vi "RT Driver VI.vi"(7 "Operation":T1, 11 "Device Reference in":T2 format="%.0x") -> (0 "Error Code":i32)   [LabVIEW 2015, in "Control Addon Engine.lvlib"]
uses:
  Control Addon Engine.lvlib
  <vilib>/NI Veristand/Custom Device API/Custom Device Item Ref.ctl
  <vilib>/NI Veristand/Custom Device API/Model Interface Driver VI Operation.ctl
  Types/RT Driver State Variables.ctl
  Types/RT Configuration.ctl
  Shared/Types/Gain Schedule.ctl
  Shared/Types/Compiled Settings.ctl
  Shared/Types/Compiled PID Settings.ctl
  <vilib>/NI Veristand/Custom Device API/Block Data Reference.ctl
  <vilib>/NI Veristand/Custom Device API/Data Reference.ctl
  Shared/Types/Compiled Industrial Settings.ctl
  Shared/Types/Compiled Industrial Parameters.ctl
  <vilib>/NI/NI VeriStand Inline Async API/_VS Inline Async API/VS Inline Async API/VS Inline Async API.lvclass
  <vilib>/NI Veristand/Custom Device API/NI VeriStand - Get Channel Values by Block Data Reference.vi
  <vilib>/addons/control/pid/pid.llb/PID Advanced (DBL Array).vi
  <vilib>/NI Veristand/Custom Device API/NI VeriStand - Set Channel Values by Block Data Reference.vi
  SubVIs/Get PID Gains from Schedule.vi
  SubVIs/Digital Debounce Filter.vi
  <vilib>/addons/control/pid/pid.llb/PID Parameter Manager (DBL Array).vi
  <vilib>/addons/control/pid/pid.llb/PID Derivative Action Buffered (DBL Array).vi
  <vilib>/addons/control/pid/pid.llb/PID Get Advanced Error (DBL Array).vi
  <vilib>/addons/control/pid/pid.llb/PID Integral Action Buffered (DBL Array).vi
  <vilib>/addons/control/pid/pid.llb/PID Resize 1D Array.vi
  <vilib>/addons/control/pid/pid.llb/PID Get Advanced Error (DBL).vi
  <vilib>/NI Veristand/Custom Device API/Global Data Refs.vi
  <vilib>/addons/control/pid/pid.llb/PID Gain Schedule.vi
  <vilib>/addons/control/pid/pid.llb/PID Gain Schedule (DBL).vi
  <vilib>/addons/control/pid/pid.llb/PID Output Rate Limiter.vi
  <vilib>/addons/control/pid/pid.llb/PID Output Rate Limiter (DBL Array).vi
  Shared/Control Addon Shared.lvlib
  <vilib>/NI VeriStand/Custom Device API/Custom Device API.lvlib
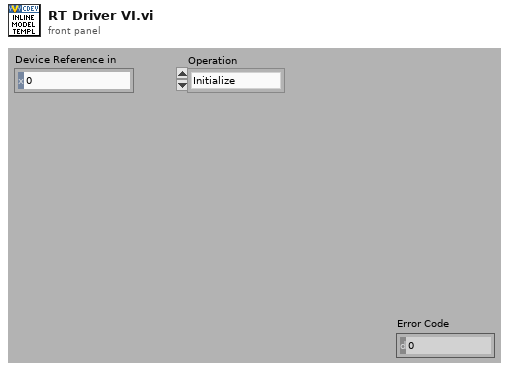
[diagram p1: front panel]
types:
  T1 = typedef "Custom Device API.lvlib/Model Interface Driver VI Operation.ctl" = enum16{"Initialize", "Start", "Execute Model", "Close"}
  T2 = typedef "Custom Device API.lvlib/Custom Device Item Ref.ctl" = u64
  T3 = typedef "Control Addon Engine.lvlib/RT Driver State Variables.ctl" = cluster{"Config":T4, "Init":bool, "Async":refnum<class "VS Inline Async API.lvclass">}
  T4 = typedef "Control Addon Engine.lvlib/RT Configuration.ctl" = cluster{"Parameter Refs":refnum<data-value>[], "Config":T5}
  T5 = typedef "Control Addon Shared.lvlib/Compiled Settings.ctl" = cluster{"PID Settings":T6, "Name":string, "Industrial Settings":T10}
  T6 = typedef "Control Addon Shared.lvlib/Compiled PID Settings.ctl" = cluster{"Gain Schedule":T7[], "Enable Live Updates":bool[], "output range":cluster{"output high":dbl, "output low":dbl}[], "setpoint range":cluster{"setpoint high":dbl, "setpoint low":dbl}[], "Write Refs":T8[], "Write Data":dbl[], "Read Refs":T8[], "Read Data":dbl[], "Control Loop Names":string[], "Enable Gain Scheduling":bool[], "Output Rate Limiter":dbl[], "dt":dbl, "setpoint high limit":dbl[], "setpoint low limit":dbl[], "output high limit":dbl[], "output low limit":dbl[]}
  T7 = typedef "Control Addon Shared.lvlib/Gain Schedule.ctl" = cluster{"Gain Schedule":cluster{"PID gains":cluster{"proportional gain (Kc)":dbl, "integral time (Ti, min)":dbl, "derivative time (Td, min)":dbl}, "max value":dbl}[]}
  T8 = typedef "Custom Device API.lvlib/Block Data Reference.ctl" = cluster{"Data Reference":T9, "Offset":u64, "Length":u64}
  T9 = typedef "Custom Device API.lvlib/Data Reference.ctl" = i32
  T10 = typedef "Control Addon Shared.lvlib/Compiled Industrial Settings.ctl" = cluster{"output range":cluster{"output high":dbl, "output low":dbl}[], "setpoint range":cluster{"setpoint high":dbl, "setpoint low":dbl}[], "Write Refs":T8[], "Write Data":dbl[], "Read Refs":T8[], "Read Data":dbl[], "Control Loop Names":string[], "Parameters":T11[], "Previous States":bool[], "Previous Counts":u64[]}
  T11 = typedef "Control Addon Shared.lvlib/Compiled Industrial Parameters.ctl" = cluster{"Enable Hysteresis":bool, "Hysteresis":dbl, "Minimum Switching":u64}
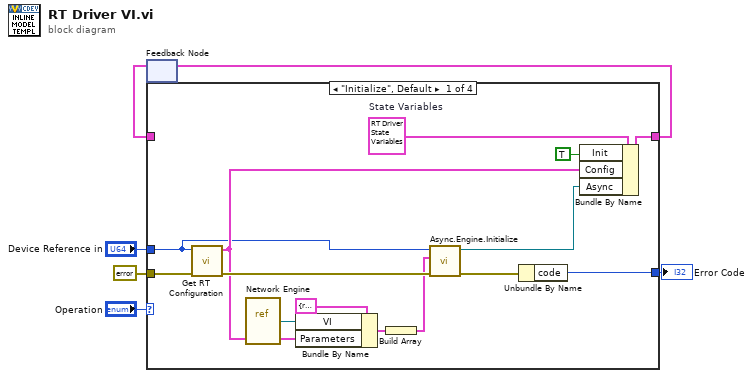
[diagram p0: block diagram]
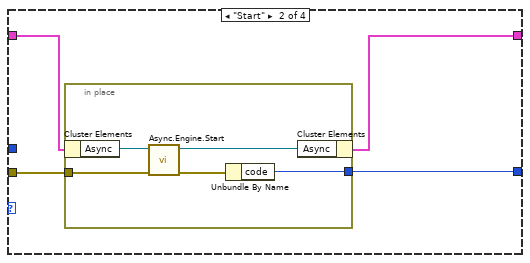
[diagram p2: hidden frame]
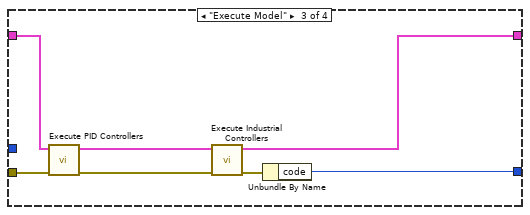
[diagram p3: hidden frame]
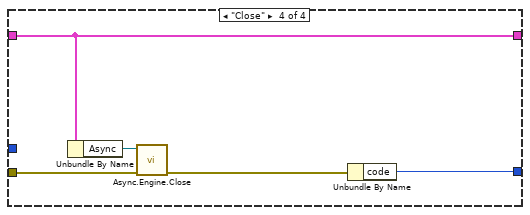
[diagram p4: hidden frame]
diagram:
  n1 = feedback #1() -> (w5:T3)  [unwired: 1 out]
  n2 = case shown="\"Initialize\", Default" "Operation" {
    tunnel: [w16 w21 w32 w41] -> w1
    tunnel: w5 -> [_ w22 w35 w41]
    tunnel: "Device Reference in" -> [w8 _ _ _]
    tunnel: [w20 w24 w33 w40] -> w3
    tunnel: errorcluster {"status"=FALSE, "code"=0, "source"=""} ("error in (no error)") -> [w19 w23 w36 w39]
    frame "Initialize", Default {
      w14 = T3 {"Config"={"Parameter Refs"=[], "Config"={"PID Settings"={"Gain Schedule"=[], "Enable Live Updates"=[], "output range"=[], "setpoint range"=[], "Write Refs"=[], "Write Data"=[], "Read Refs"=[], "Read Data"=[], "Control Loop Names"=[], "Enable Gain Scheduling"=[], "Output Rate Limiter"=[], "dt"=0.0, "setpoint high limit"=[], "setpoint low limit"=[], "output high limit"=[], "output low limit"=[]}, "Name"="", "Industrial Settings"={"output range"=[], "setpoint range"=[], "Write Refs"=[], "Write Data"=[], "Read Refs"=[], "Read Data"=[], "Control Loop Names"=[], "Parameters"=[], "Previous States"=[], "Previous Counts"=[]}}}, "Init"=FALSE, "Async"=refnum}  # State Variables
      n3 = call "Get RT Configuration.vi"("error in (no error)"=w19, "Device Reference in"=w8) -> ("error out"=w18:errorcluster, "RT Config"=w11:T4)  [unwired: 8 in]
      n4 = vi-ref "Network Engine.vi"() -> (w12:refnum<vi>)
      n5 = Bundle By Name(cluster=cluster{"VI":refnum<vi>, "Parameters":variant} {"VI"=refnum, "Parameters"=variant} ("Process"), "VI"=w12, "Parameters"=w11) -> (w10:cluster{"VI":refnum<vi>, "Parameters":variant})
      n6 = Build Array(w10) -> (w9:cluster{"VI":refnum<vi>, "Parameters":variant}[])
      n7 = call <vilib>:"Async.Engine.Initialize.vi"("error in (no error)"=w18, "Processes"=w9, "Custom Device Ref"=w8) -> ("error out"=w17:errorcluster, "Async"=w7:refnum<class "VS Inline Async API.lvclass">)  [unwired: 7 in]
      n8 = Unbundle By Name(w17) -> ("code"=w20:i32)
      n9 = Bundle By Name(cluster=w14, "Init"=TRUE, "Config"=w11, "Async"=w7) -> (w16:T3)
    }
    frame "Start" {
      n10 = in-place {
        in-place-border: [w29] -> w24
        in-place-border: w23 -> [w28]
        n11 = in-place-cluster #2(w22) -> ("Async"=w26:refnum<class "VS Inline Async API.lvclass">)
        n12 = call <vilib>:"Async.Engine.Start.vi"("error in (no error)"=w28, "VS Inline Async API in"=w26) -> ("error out"=w27:errorcluster, "VS Inline Async API out"=w25:refnum<class "VS Inline Async API.lvclass">)  [unwired: 8 in]
        n13 = Unbundle By Name(w27) -> ("code"=w29:i32)
        n14 = in-place-cluster #2("Async"=w25) -> (w21:T3)
      }
    }
    frame "Execute Model" {
      n15 = call "Execute PID Controllers.vi"("error in (no error)"=w36, "State Variables in"=w35) -> ("error out"=w31:errorcluster, "State Variables out"=w34:T3)  [unwired: 8 in]
      n16 = call "Execute Industrial Controllers.vi"("error in (no error)"=w31, "State Variables in"=w34) -> ("error out"=w30:errorcluster, "State Variables out"=w32:T3)  [unwired: 8 in]
      n17 = Unbundle By Name(w30) -> ("code"=w33:i32)
    }
    frame "Close" {
      n18 = Unbundle By Name(w41) -> ("Async"=w37:refnum<class "VS Inline Async API.lvclass">)
      n19 = call <vilib>:"Async.Engine.Close.vi"("error in (no error)"=w39, "Async in"=w37) -> ("error out"=w38:errorcluster)  [unwired: 8 in, 1 out]
      n20 = Unbundle By Name(w38) -> ("code"=w40:i32)
    }
  }
  "Error Code" <- w3
  n21 = feedback-in #1(w1) -> ()
